vi "Defaults.vi"(8 "error in (no error)":errorcluster, 11 "MB Slave in":refnum<class "iC7-DCDC.lvclass">) -> (0 "error out":errorcluster, 3 "MB Slave out":refnum<class "iC7-DCDC.lvclass">)   [LabVIEW 2021, in "iC7-DCDC.lvclass"]
uses:
  iC7-DCDC.lvclass
  C:/Program Files (x86)/National Instruments/LabVIEW 2021/user.lib/S2 Labs/Module Framework/Modules/Modbus/Modbus Slave Base/Modbus Slave Base.lvclass
  <userlib>/S2 Labs/Modbus Toolkit/TypeDefs/MB Element.ctl
  <userlib>/S2 Labs/Modbus Toolkit/TypeDefs/Endianness Type.ctl
  <userlib>/S2 Labs/Modbus Toolkit/TypeDefs/Access Type.ctl
  <userlib>/S2 Labs/Module Framework/Modules/Modbus/Modbus Slave Base/Modbus Slave Base.lvclass/Modbus Slave Base.ctl
  <userlib>/S2 Labs/Module Framework/Modules/Modbus/Modbus Slave Base/Write MB Map.vi
  MB Slave Simulator Base/MB Slave Simulator Base.lvclass
  <userlib>/S2 Labs/Modbus Toolkit/S2L Modbus API.lvclass
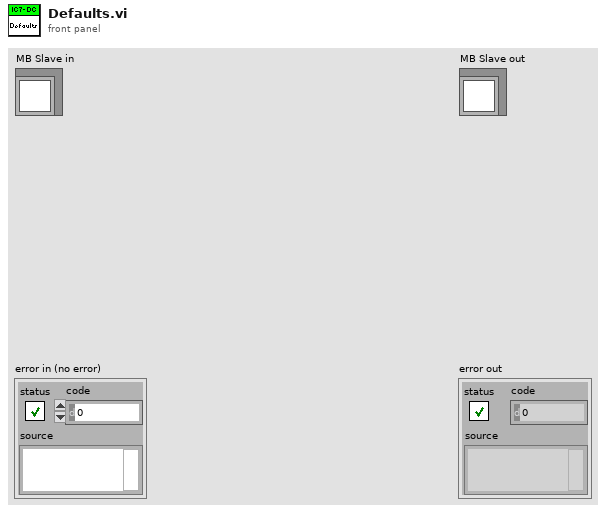
[diagram p1: front panel]
types:
  T1 = typedef "S2L Modbus API.lvclass/MB Element.ctl" = cluster{"Label":string, "Prefix":u8, "Address":u16, "Datatype":string, "Register Count":u8, "Multiplier":dbl, "Offset":dbl, "Unit":string, "Endianness":T2, "Access":T3, "LUT":string[], "Poll Rate(ms)":u16, "Mapping":cluster{"Module":string, "Channel":string}}
  T2 = typedef "Endianness Type.ctl" = enum16{"Big-Endian", "Little-Endian", "Big-Endian Byte Swap", "Little-Endian Byte Swap"}
  T3 = typedef "S2L Modbus API.lvclass/Access Type.ctl" = enum16{"R/W", "R", "W"}
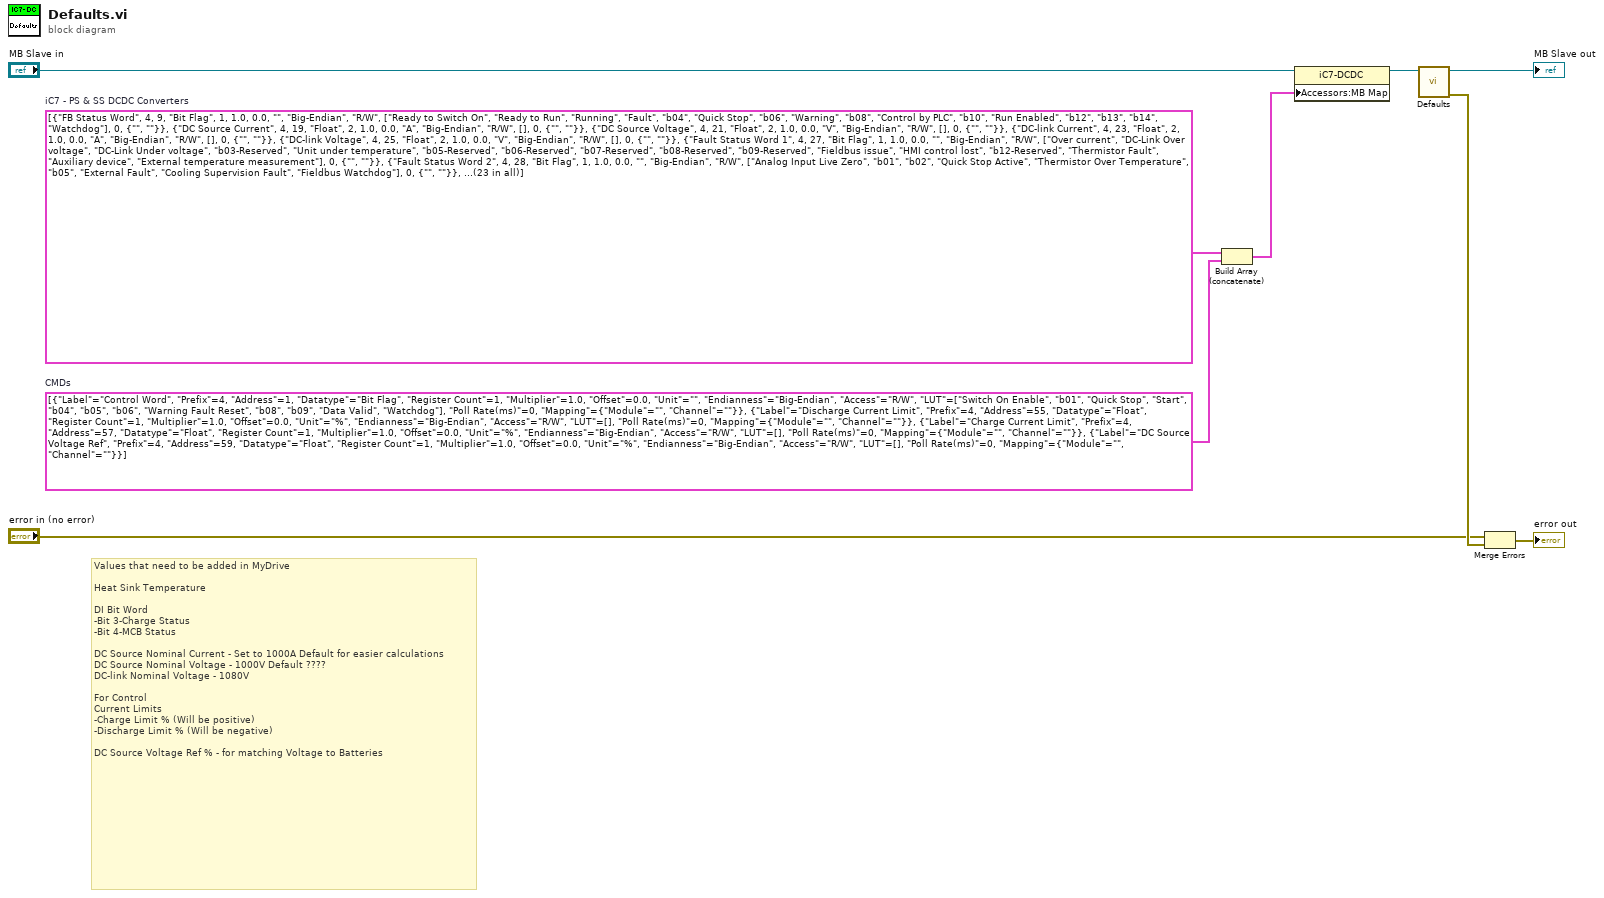
[diagram p0: block diagram]
diagram:
  w3 = T1[] [{"Label"="Control Word", "Prefix"=4, "Address"=1, "Datatype"="Bit Flag", "Register Count"=1, "Multiplier"=1.0, "Offset"=0.0, "Unit"="", "Endianness"=enum."Big-Endian", "Access"=enum."R/W", "LUT"=["Switch On Enable", "b01", "Quick Stop", "Start", "b04", "b05", "b06", "Warning Fault Reset", "b08", "b09", "Data Valid", "Watchdog"], "Poll Rate(ms)"=0, "Mapping"={"Module"="", "Channel"=""}}, {"Label"="Discharge Current Limit", "Prefix"=4, "Address"=55, "Datatype"="Float", "Register Count"=1, "Multiplier"=1.0, "Offset"=0.0, "Unit"="%", "Endianness"=enum."Big-Endian", "Access"=enum."R/W", "LUT"=[], "Poll Rate(ms)"=0, "Mapping"={"Module"="", "Channel"=""}}, {"Label"="Charge Current Limit", "Prefix"=4, "Address"=57, "Datatype"="Float", "Register Count"=1, "Multiplier"=1.0, "Offset"=0.0, "Unit"="%", "Endianness"=enum."Big-Endian", "Access"=enum."R/W", "LUT"=[], "Poll Rate(ms)"=0, "Mapping"={"Module"="", "Channel"=""}}, {"Label"="DC Source Voltage Ref", "Prefix"=4, "Address"=59, "Datatype"="Float", "Register Count"=1, "Multiplier"=1.0, "Offset"=0.0, "Unit"="%", "Endianness"=enum."Big-Endian", "Access"=enum."R/W", "LUT"=[], "Poll Rate(ms)"=0, "Mapping"={"Module"="", "Channel"=""}}]  # CMDs
  w2 = T1[] [{"Label"="FB Status Word", "Prefix"=4, "Address"=9, "Datatype"="Bit Flag", "Register Count"=1, "Multiplier"=1.0, "Offset"=0.0, "Unit"="", "Endianness"=enum."Big-Endian", "Access"=enum."R/W", "LUT"=["Ready to Switch On", "Ready to Run", "Running", "Fault", "b04", "Quick Stop", "b06", "Warning", "b08", "Control by PLC", "b10", "Run Enabled", "b12", "b13", "b14", "Watchdog"], "Poll Rate(ms)"=0, "Mapping"={"Module"="", "Channel"=""}}, {"Label"="DC Source Current", "Prefix"=4, "Address"=19, "Datatype"="Float", "Register Count"=2, "Multiplier"=1.0, "Offset"=0.0, "Unit"="A", "Endianness"=enum."Big-Endian", "Access"=enum."R/W", "LUT"=[], "Poll Rate(ms)"=0, "Mapping"={"Module"="", "Channel"=""}}, {"Label"="DC Source Voltage", "Prefix"=4, "Address"=21, "Datatype"="Float", "Register Count"=2, "Multiplier"=1.0, "Offset"=0.0, "Unit"="V", "Endianness"=enum."Big-Endian", "Access"=enum."R/W", "LUT"=[], "Poll Rate(ms)"=0, "Mapping"={"Module"="", "Channel"=""}}, {"Label"="DC-link Current", "Prefix"=4, "Address"=23, "Datatype"="Float", "Register Count"=2, "Multiplier"=1.0, "Offset"=0.0, "Unit"="A", "Endianness"=enum."Big-Endian", "Access"=enum."R/W", "LUT"=[], "Poll Rate(ms)"=0, "Mapping"={"Module"="", "Channel"=""}}, {"Label"="DC-link Voltage", "Prefix"=4, "Address"=25, "Datatype"="Float", "Register Count"=2, "Multiplier"=1.0, "Offset"=0.0, "Unit"="V", "Endianness"=enum."Big-Endian", "Access"=enum."R/W", "LUT"=[], "Poll Rate(ms)"=0, "Mapping"={"Module"="", "Channel"=""}}, {"Label"="Fault Status Word 1", "Prefix"=4, "Address"=27, "Datatype"="Bit Flag", "Register Count"=1, "Multiplier"=1.0, "Offset"=0.0, "Unit"="", "Endianness"=enum."Big-Endian", "Access"=enum."R/W", "LUT"=["Over current", "DC-Link Over voltage", "DC-Link Under voltage", "b03-Reserved", "Unit under temperature", "b05-Reserved", "b06-Reserved", "b07-Reserved", "b08-Reserved", "b09-Reserved", "Fieldbus issue", "HMI control lost", "b12-Reserved", "Thermistor Fault", "Auxiliary device", "External temperature measurement"], "Poll Rate(ms)"=0, "Mapping"={"Module"="", "Channel"=""}}, {"Label"="Fault Status Word 2", "Prefix"=4, "Address"=28, "Datatype"="Bit Flag", "Register Count"=1, "Multiplier"=1.0, "Offset"=0.0, "Unit"="", "Endianness"=enum."Big-Endian", "Access"=enum."R/W", "LUT"=["Analog Input Live Zero", "b01", "b02", "Quick Stop Active", "Thermistor Over Temperature", "b05", "External Fault", "Cooling Supervision Fault", "Fieldbus Watchdog"], "Poll Rate(ms)"=0, "Mapping"={"Module"="", "Channel"=""}}, {"Label"="Warning Status Word 1", "Prefix"=4, "Address"=29, "Datatype"="Bit Flag", "Register Count"=1, "Multiplier"=1.0, "Offset"=0.0, "Unit"="", "Endianness"=enum."Big-Endian", "Access"=enum."R/W", "LUT"=["Over current", "DC-Link Over voltage", "DC-Link Under voltage", "b03-Reserved", "Unit under temperature ", "b05-Reserved", "b06-Reserved", "b07-Reserved", "Earth Warning", "b09-Reserved", "Fieldbus issue", "HMI control lost", "b12-Reserved", "Thermistor Warning", "Auxiliary device", "External temperature measurement"], "Poll Rate(ms)"=0, "Mapping"={"Module"="", "Channel"=""}}, {"Label"="Warning Status Word 2", "Prefix"=4, "Address"=30, "Datatype"="Bit Flag", "Register Count"=1, "Multiplier"=1.0, "Offset"=0.0, "Unit"="", "Endianness"=enum."Big-Endian", "Access"=enum."R/W", "LUT"=["Analog Input Live Zero", "b01-Reserved", "b02-Reserved", "Quick Stop Active", "Thermistor Over Temperature", "b05-Reserved", "External Warning", "Cooling Supervision Warning", "Fieldbus Watchdog"], "Poll Rate(ms)"=0, "Mapping"={"Module"="", "Channel"=""}}, {"Label"="Last Fault Number", "Prefix"=4, "Address"=31, "Datatype"="U16", "Register Count"=1, "Multiplier"=1.0, "Offset"=0.0, "Unit"="", "Endianness"=enum."Big-Endian", "Access"=enum."R/W", "LUT"=[], "Poll Rate(ms)"=0, "Mapping"={"Module"="", "Channel"=""}}, {"Label"="Last Warning Number", "Prefix"=4, "Address"=32, "Datatype"="U16", "Register Count"=1, "Multiplier"=1.0, "Offset"=0.0, "Unit"="", "Endianness"=enum."Big-Endian", "Access"=enum."R/W", "LUT"=[], "Poll Rate(ms)"=0, "Mapping"={"Module"="", "Channel"=""}}, {"Label"="DCDC Control Status Word", "Prefix"=4, "Address"=33, "Datatype"="Bit Flag", "Register Count"=1, "Multiplier"=1.0, "Offset"=0.0, "Unit"="", "Endianness"=enum."Big-Endian", "Access"=enum."R/W", "LUT"=["Converter Control Ready", "Running", "b02-Reserved", "Fault Active", "b04-Reserved", "b05-Reserved", "DC-link Charged"], "Poll Rate(ms)"=0, "Mapping"={"Module"="", "Channel"=""}}, {"Label"="FB DC-link Voltage Ref", "Prefix"=4, "Address"=34, "Datatype"="Float", "Register Count"=1, "Multiplier"=1.0, "Offset"=0.0, "Unit"="%", "Endianness"=enum."Big-Endian", "Access"=enum."R/W", "LUT"=[], "Poll Rate(ms)"=0, "Mapping"={"Module"="", "Channel"=""}}, {"Label"="FB DC-link Current Ref", "Prefix"=4, "Address"=36, "Datatype"="Float", "Register Count"=1, "Multiplier"=1.0, "Offset"=0.0, "Unit"="%", "Endianness"=enum."Big-Endian", "Access"=enum."R/W", "LUT"=[], "Poll Rate(ms)"=0, "Mapping"={"Module"="", "Channel"=""}}, {"Label"="FB DC Source Voltage Ref", "Prefix"=4, "Address"=38, "Datatype"="Float", "Register Count"=1, "Multiplier"=1.0, "Offset"=0.0, "Unit"="%", "Endianness"=enum."Big-Endian", "Access"=enum."R/W", "LUT"=[], "Poll Rate(ms)"=0, "Mapping"={"Module"="", "Channel"=""}}, {"Label"="FB DC Source Current Ref", "Prefix"=4, "Address"=40, "Datatype"="Float", "Register Count"=1, "Multiplier"=1.0, "Offset"=0.0, "Unit"="%", "Endianness"=enum."Big-Endian", "Access"=enum."R/W", "LUT"=[], "Poll Rate(ms)"=0, "Mapping"={"Module"="", "Channel"=""}}, {"Label"="X52 Voltage Measurement", "Prefix"=4, "Address"=42, "Datatype"="Float", "Register Count"=1, "Multiplier"=1.0, "Offset"=0.0, "Unit"="V", "Endianness"=enum."Big-Endian", "Access"=enum."R/W", "LUT"=[], "Poll Rate(ms)"=0, "Mapping"={"Module"="", "Channel"=""}}, {"Label"="X53 Voltage Measurement", "Prefix"=4, "Address"=44, "Datatype"="Float", "Register Count"=1, "Multiplier"=1.0, "Offset"=0.0, "Unit"="V", "Endianness"=enum."Big-Endian", "Access"=enum."R/W", "LUT"=[], "Poll Rate(ms)"=0, "Mapping"={"Module"="", "Channel"=""}}, {"Label"="Heat Sink Temperature", "Prefix"=4, "Address"=46, "Datatype"="Float", "Register Count"=1, "Multiplier"=1.0, "Offset"=0.0, "Unit"="C", "Endianness"=enum."Big-Endian", "Access"=enum."R/W", "LUT"=[], "Poll Rate(ms)"=0, "Mapping"={"Module"="", "Channel"=""}}, {"Label"="DI Bit Word", "Prefix"=4, "Address"=48, "Datatype"="Bit Flag", "Register Count"=1, "Multiplier"=1.0, "Offset"=0.0, "Unit"="", "Endianness"=enum."Big-Endian", "Access"=enum."R/W", "LUT"=["b00", "b01", "b02", "Breaker Charged", "MCB Feedback"], "Poll Rate(ms)"=0, "Mapping"={"Module"="", "Channel"=""}}, {"Label"="DC Source Nominal Current", "Prefix"=4, "Address"=49, "Datatype"="Float", "Register Count"=1, "Multiplier"=1.0, "Offset"=0.0, "Unit"="A", "Endianness"=enum."Big-Endian", "Access"=enum."R/W", "LUT"=[], "Poll Rate(ms)"=0, "Mapping"={"Module"="", "Channel"=""}}, {"Label"="DC Source Nominal Voltage", "Prefix"=4, "Address"=51, "Datatype"="Float", "Register Count"=1, "Multiplier"=1.0, "Offset"=0.0, "Unit"="V", "Endianness"=enum."Big-Endian", "Access"=enum."R/W", "LUT"=[], "Poll Rate(ms)"=0, "Mapping"={"Module"="", "Channel"=""}}, {"Label"="DC-link Nominal Voltage", "Prefix"=4, "Address"=53, "Datatype"="Float", "Register Count"=1, "Multiplier"=1.0, "Offset"=0.0, "Unit"="V", "Endianness"=enum."Big-Endian", "Access"=enum."R/W", "LUT"=[], "Poll Rate(ms)"=0, "Mapping"={"Module"="", "Channel"=""}}]  # iC7 - PS & SS DCDC Converters
  # "Values that need to be added in MyDrive\n\nHeat Sink Temperature\n\nDI Bit Word \n-Bit 3-Charge Status\n-Bit 4-MCB Status\n\nDC Source Nominal Current - Set to 1000A Default for easier calculations\nDC Source Nominal Voltage - 1000V Default ????\nDC-link Nominal Voltage - 1080V\n\nFor Control\nCurrent Limits\n-Charge Limit % (Will be positive)\n-Discharge Limit % (Will be negative)\n\nDC Source Voltage Ref % - for matching Voltage to Batteries"
  n1 = Build Array (concatenate)(w2, w3) -> (w1:T1[])
  n2 = property class="iC7-DCDC"(reference="MB Slave in", "Accessors:MB Map"=w1) -> (reference out=w4:refnum<class "iC7-DCDC.lvclass">)  [unwired: 1 in, 1 out]
  n3 = call-parent "Defaults.vi"("MB Slave in"=w4) -> ("error out"=w8:errorcluster, "MB Slave out"=→"MB Slave out":refnum<class "iC7-DCDC.lvclass">)  [unwired: 9 in]
  n4 = Merge Errors("error in (no error)", w8) -> (→"error out":errorcluster)
